vi "rolling game.vi"() -> ()   [LabVIEW 2014]
panel:
  out "Waveform Chart":cluster{dbl, dbl, dbl}(graph)
  out "player2 win rate":dbl
  out "tie rate":dbl
  out "a":dbl
  out "0:tie\n1:player1 win\n-1:player2 win":dbl
  out "player 2":dbl
  out "player1":dbl
  in  "roll":bool
  # "player1 win rate"
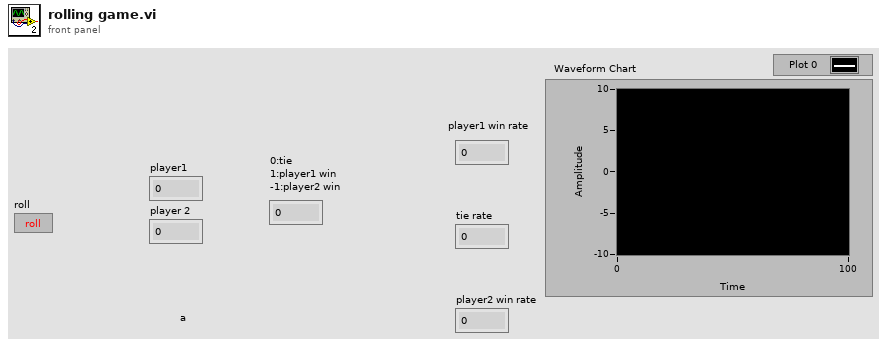
[diagram p1: front panel]
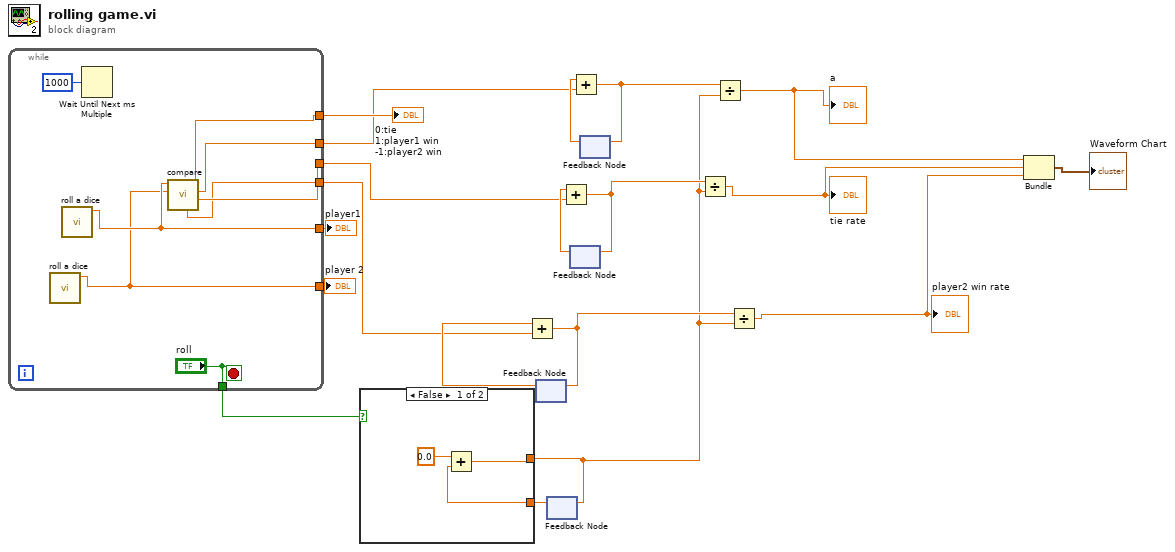
[diagram p0: block diagram]
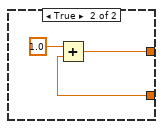
[diagram p2: hidden frame]
diagram:
  n1 = while {
    tunnel: [w26] -> w18
    tunnel: [w25] -> w19
    tunnel: [w24] -> w17
    tunnel: [w23] -> w15
    tunnel: [w22] -> w13
    tunnel: [w21] -> w11
    tunnel: ["roll"] -> w10
    stop <- "roll" stop-if-true
    n2 = call "roll a dice.vi"() -> ("Numeric"=w25:dbl)  [unwired: 11 in]
    n3 = call "roll a dice.vi"() -> ("Numeric"=w26:dbl)  [unwired: 11 in]
    n4 = Wait Until Next ms Multiple(millisecond multiple=u32 1000) -> ()  [unwired: 1 out]
    n5 = call "compare.vi"("input variable 2"=w25, "input variable"=w26) -> ("b"=w22:dbl, "a"=w23:dbl, "z"=w24:dbl, "c"=w21:dbl)  [unwired: 6 in]
  }
  "player1" <- w18
  "player 2" <- w19
  "0:tie\n1:player1 win\n-1:player2 win" <- w17
  n6 = feedback #1() -> (w12:dbl)  [unwired: 1 in]
  n7 = Add(x=w12, y=w11) -> (x+y=w6:dbl)
  n8 = feedback-in #1(w6) -> ()
  n9 = feedback #2() -> (w9:dbl)  [unwired: 1 in]
  n10 = case shown="False" w10 {
    tunnel: [w29 w33] -> w5
    tunnel: w9 -> [w28 w31]
    frame False {
      n11 = Add(x=0.0, y=w28) -> (x+y=w29:dbl)
    }
    frame True {
      n12 = Add(x=1.0, y=w31) -> (x+y=w33:dbl)
    }
  }
  n13 = feedback-in #2(w5) -> ()
  n14 = feedback #3() -> (w14:dbl)  [unwired: 1 in]
  n15 = Add(x=w14, y=w13) -> (x+y=w7:dbl)
  n16 = feedback-in #3(w7) -> ()
  n17 = feedback #4() -> (w16:dbl)  [unwired: 1 in]
  n18 = Add(x=w16, y=w15) -> (x+y=w8:dbl)
  n19 = feedback-in #4(w8) -> ()
  n20 = Divide(x=w7, y=w5) -> (x/y=w3:dbl)
  "tie rate" <- w3
  n21 = Divide(x=w8, y=w5) -> (x/y=w4:dbl)
  "a" <- w4
  n22 = Divide(x=w6, y=w5) -> (x/y=w2:dbl)
  "player2 win rate" <- w2
  n23 = Bundle(w4, w3, w2) -> (→"Waveform Chart":cluster{dbl, dbl, dbl})  [unwired: 1 in]
